vi "_ReplaceInfoString.vi"(5 "Value":string, 6 "Key":string, 7 "SystemInfo":string="Instrument Model: IONICS 3Q 220\nInstrument Secrial Number: A2103536\nManufacturer: IONICS MASS SPECTROMETRY\nScan Mode: Q1, Positive\nResolution: Unit_Unit\nSource: ESI2\nMethod: +Q1 PPG\nCurrent Detector (V): 2500\nOptimized Detector (V): 2600") -> (3 "SystemInfoOut":string)   [LabVIEW 2015]
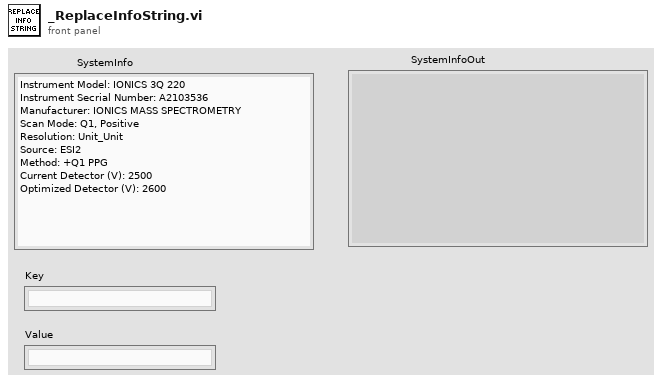
[diagram p1: front panel]
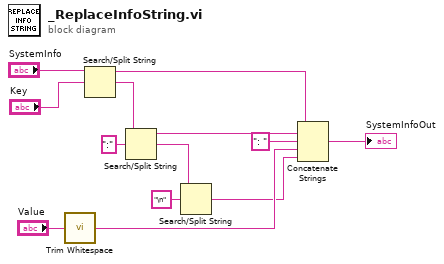
[diagram p0: block diagram]
diagram:
  n1 = call <vilib>:"Trim Whitespace.vi"("string"="Value") -> ("trimmed string"=w3:string)  [unwired: 1 in]
  n2 = Search/Split String(string="SystemInfo", search string/char (-)="Key") -> (substring before match=w6:string, match + rest of string=w10:string)  [unwired: 1 in, 1 out]
  n3 = Search/Split String(string=w10, search string/char (-)=":") -> (substring before match=w5:string, match + rest of string=w7:string)  [unwired: 1 in, 1 out]
  n4 = Search/Split String(string=w7, search string/char (-)="\n") -> (match + rest of string=w2:string)  [unwired: 1 in, 2 out]
  n5 = Concatenate Strings(w6, w5, ": " ("search string/char (-)"), w3, w2) -> (→"SystemInfoOut":string)
